vi "HandleObs.vi"(8 "error in (no error)":errorcluster, 11 "S4GUI in":refnum<class "S4GUI.lvclass">) -> (0 "error out":errorcluster, 3 "S4GUI out":refnum<class "S4GUI.lvclass">)   [LabVIEW 2018, in "S4GUI.lvclass"]
uses:
  S4GUI.lvclass
  S4GUI.lvclass/S4GUI.ctl
  Acquisition/Acquisition.lvclass
  Channel/Channel.lvclass
  StateMachine/State Machine.lvclass
  SyncBox/Sync Box.lvclass
  Trigger/Trigger.lvclass
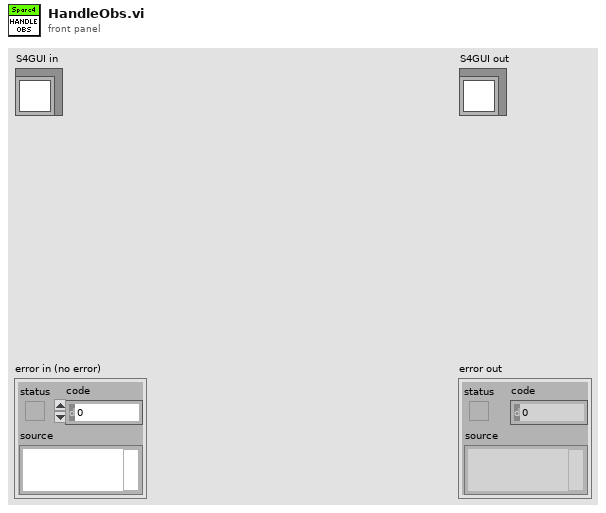
[diagram p1: front panel]
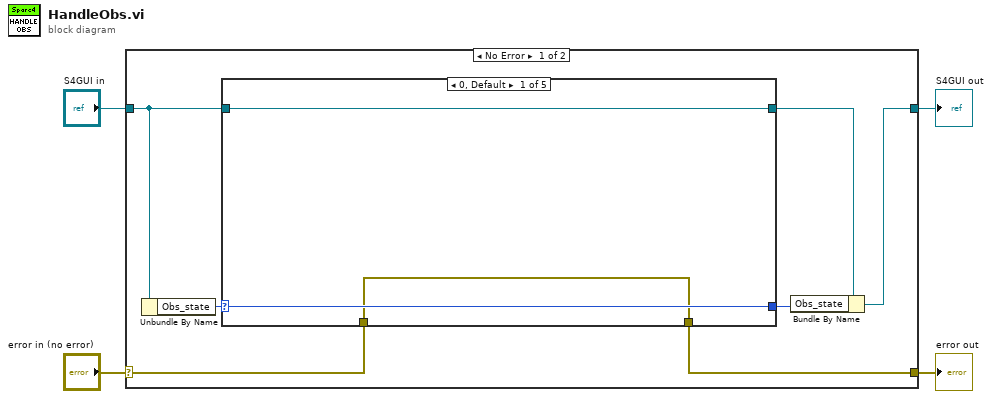
[diagram p0: block diagram]
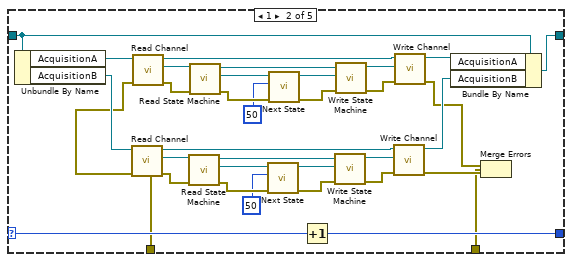
[diagram p2: hidden frame]
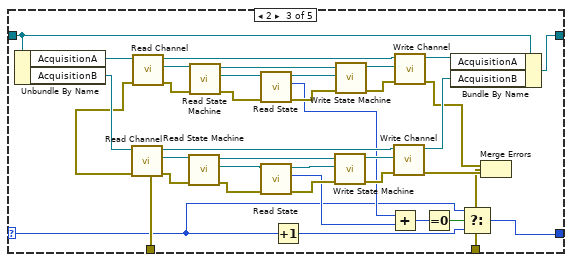
[diagram p3: hidden frame]
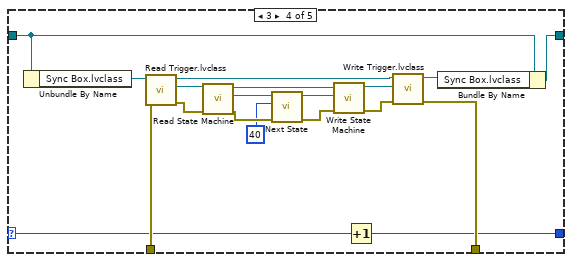
[diagram p4: hidden frame]
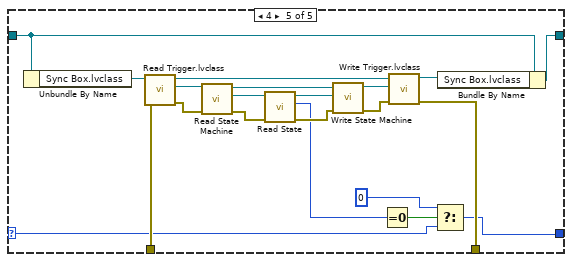
[diagram p5: hidden frame]
diagram:
  n1 = case shown="No Error" "error in (no error)" {
    selector: "error in (no error)" -> [w6 w127]
    tunnel: [w5 w127] -> w3
    tunnel: [w7 w126] -> w1
    tunnel: "S4GUI in" -> [w11 w126]
    frame No Error {
      n2 = Unbundle By Name(w11) -> ("Obs_state"=w10:u32)
      n3 = case shown="0, Default" w10 {
        selector: w10 -> [w14 w46 w49 w87 w109]
        tunnel: [w12 w48 w85 w104 w125] -> w9
        tunnel: w11 -> [w12 w47 w84 w103 w124]
        tunnel: [w14 w45 w50 w86 w105] -> w8
        tunnel: w6 -> [w13 w18 w67 w99 w120]
        tunnel: [w13 w15 w64 w98 w119] -> w5
        frame 0, Default {
        }
        frame 1 {
          n4 = Unbundle By Name(w47) -> ("AcquisitionA"=w44:refnum<class "Acquisition.lvclass">, "AcquisitionB"=w20:refnum<class "Acquisition.lvclass">)
          n5 = call-dynamic "Read Channel.vi"("error in (no error)"=w18, "Acquisition in"=w20) -> ("error out"=w30:errorcluster, "Channel.lvclass"=w29:refnum<class "Channel.lvclass">, "Acquisition out"=w31:refnum<class "Acquisition.lvclass">)  [unwired: 7 in]
          n6 = call-dynamic "Read Channel.vi"("error in (no error)"=w18, "Acquisition in"=w44) -> ("error out"=w41:errorcluster, "Channel.lvclass"=w40:refnum<class "Channel.lvclass">, "Acquisition out"=w42:refnum<class "Acquisition.lvclass">)  [unwired: 7 in]
          n7 = call-dynamic "Read State Machine.vi"("error in (no error)"=w30, "Device in"=w29) -> ("error out"=w25:errorcluster, "State Machine.lvclass"=w23:refnum<class "State Machine.lvclass">, "Device out"=w28:refnum<class "Channel.lvclass">)  [unwired: 7 in]
          n8 = call-dynamic "Read State Machine.vi"("error in (no error)"=w41, "Device in"=w40) -> ("error out"=w36:errorcluster, "State Machine.lvclass"=w34:refnum<class "State Machine.lvclass">, "Device out"=w39:refnum<class "Channel.lvclass">)  [unwired: 7 in]
          n9 = call "Next State.vi"("error in (no error)"=w25, "New_State"=50, "State Machine in"=w23) -> ("error out"=w21:errorcluster, "State Machine out"=w22:refnum<class "State Machine.lvclass">)  [unwired: 7 in]
          n10 = call "Next State.vi"("error in (no error)"=w36, "New_State"=50, "State Machine in"=w34) -> ("error out"=w32:errorcluster, "State Machine out"=w33:refnum<class "State Machine.lvclass">)  [unwired: 7 in]
          n11 = Increment(x=w46) -> (x+1=w45:u32)
          n12 = call-dynamic "Write State Machine.vi"("error in (no error)"=w21, "State Machine.lvclass"=w22, "Device in"=w28) -> ("error out"=w26:errorcluster, "Device out"=w27:refnum<class "Channel.lvclass">)  [unwired: 7 in]
          n13 = call-dynamic "Write State Machine.vi"("error in (no error)"=w32, "State Machine.lvclass"=w33, "Device in"=w39) -> ("error out"=w37:errorcluster, "Device out"=w38:refnum<class "Channel.lvclass">)  [unwired: 7 in]
          n14 = call-dynamic "Write Channel.vi"("error in (no error)"=w26, "Channel.lvclass"=w27, "Acquisition in"=w31) -> ("error out"=w16:errorcluster, "Acquisition out"=w19:refnum<class "Acquisition.lvclass">)  [unwired: 7 in]
          n15 = call-dynamic "Write Channel.vi"("error in (no error)"=w37, "Channel.lvclass"=w38, "Acquisition in"=w42) -> ("error out"=w17:errorcluster, "Acquisition out"=w43:refnum<class "Acquisition.lvclass">)  [unwired: 7 in]
          n16 = Bundle By Name(cluster=w47, "AcquisitionA"=w43, "AcquisitionB"=w19) -> (w48:refnum<class "S4GUI.lvclass">)
          n17 = Merge Errors(w17, w16) -> (w15:errorcluster)
        }
        frame 2 {
          n18 = Unbundle By Name(w84) -> ("AcquisitionA"=w83:refnum<class "Acquisition.lvclass">, "AcquisitionB"=w69:refnum<class "Acquisition.lvclass">)
          n19 = call-dynamic "Read Channel.vi"("error in (no error)"=w67, "Acquisition in"=w69) -> ("error out"=w74:errorcluster, "Channel.lvclass"=w73:refnum<class "Channel.lvclass">, "Acquisition out"=w75:refnum<class "Acquisition.lvclass">)  [unwired: 7 in]
          n20 = call-dynamic "Read Channel.vi"("error in (no error)"=w67, "Acquisition in"=w83) -> ("error out"=w80:errorcluster, "Channel.lvclass"=w79:refnum<class "Channel.lvclass">, "Acquisition out"=w81:refnum<class "Acquisition.lvclass">)  [unwired: 7 in]
          n21 = call-dynamic "Read State Machine.vi"("error in (no error)"=w74, "Device in"=w73) -> ("error out"=w57:errorcluster, "State Machine.lvclass"=w61:refnum<class "State Machine.lvclass">, "Device out"=w72:refnum<class "Channel.lvclass">)  [unwired: 7 in]
          n22 = call-dynamic "Read State Machine.vi"("error in (no error)"=w80, "Device in"=w79) -> ("error out"=w59:errorcluster, "State Machine.lvclass"=w63:refnum<class "State Machine.lvclass">, "Device out"=w78:refnum<class "Channel.lvclass">)  [unwired: 7 in]
          n23 = call-dynamic "Read State.vi"("error in (no error)"=w59, "State Machine in"=w63) -> ("error out"=w58:errorcluster, "State"=w55:i32, "State Machine out"=w62:refnum<class "State Machine.lvclass">)  [unwired: 7 in]
          n24 = call-dynamic "Read State.vi"("error in (no error)"=w57, "State Machine in"=w61) -> ("error out"=w56:errorcluster, "State"=w54:i32, "State Machine out"=w60:refnum<class "State Machine.lvclass">)  [unwired: 7 in]
          n25 = Increment(x=w49) -> (x+1=w51:u32)
          n26 = call-dynamic "Write State Machine.vi"("error in (no error)"=w56, "State Machine.lvclass"=w60, "Device in"=w72) -> ("error out"=w70:errorcluster, "Device out"=w71:refnum<class "Channel.lvclass">)  [unwired: 7 in]
          n27 = call-dynamic "Write State Machine.vi"("error in (no error)"=w58, "State Machine.lvclass"=w62, "Device in"=w78) -> ("error out"=w76:errorcluster, "Device out"=w77:refnum<class "Channel.lvclass">)  [unwired: 7 in]
          n28 = Add(x=w55, y=w54) -> (x+y=w53:i32)
          n29 = call-dynamic "Write Channel.vi"("error in (no error)"=w70, "Channel.lvclass"=w71, "Acquisition in"=w75) -> ("error out"=w65:errorcluster, "Acquisition out"=w68:refnum<class "Acquisition.lvclass">)  [unwired: 7 in]
          n30 = call-dynamic "Write Channel.vi"("error in (no error)"=w76, "Channel.lvclass"=w77, "Acquisition in"=w81) -> ("error out"=w66:errorcluster, "Acquisition out"=w82:refnum<class "Acquisition.lvclass">)  [unwired: 7 in]
          n31 = Equal To 0?(x=w53) -> (x = 0?=w52:bool)
          n32 = Bundle By Name(cluster=w84, "AcquisitionA"=w82, "AcquisitionB"=w68) -> (w85:refnum<class "S4GUI.lvclass">)
          n33 = Select(t=w49, s=w52, f=w51) -> (s? t:f=w50:u32)
          n34 = Merge Errors(w66, w65) -> (w64:errorcluster)
        }
        frame 3 {
          n35 = Unbundle By Name(w103) -> ("Sync Box.lvclass"=w102:refnum<class "Sync Box.lvclass">)
          n36 = call-dynamic "Read Trigger.lvclass.vi"("error in (no error)"=w99, "Sync Box in"=w102) -> ("error out"=w97:errorcluster, "Trigger.lvclass"=w96:refnum<class "Trigger.lvclass">, "Sync Box out"=w100:refnum<class "Sync Box.lvclass">)  [unwired: 7 in]
          n37 = call-dynamic "Read State Machine.vi"("error in (no error)"=w97, "Device in"=w96) -> ("error out"=w92:errorcluster, "State Machine.lvclass"=w90:refnum<class "State Machine.lvclass">, "Device out"=w95:refnum<class "Trigger.lvclass">)  [unwired: 7 in]
          n38 = call "Next State.vi"("error in (no error)"=w92, "New_State"=40, "State Machine in"=w90) -> ("error out"=w88:errorcluster, "State Machine out"=w89:refnum<class "State Machine.lvclass">)  [unwired: 7 in]
          n39 = call-dynamic "Write State Machine.vi"("error in (no error)"=w88, "State Machine.lvclass"=w89, "Device in"=w95) -> ("error out"=w93:errorcluster, "Device out"=w94:refnum<class "Trigger.lvclass">)  [unwired: 7 in]
          n40 = Increment(x=w87) -> (x+1=w86:u32)
          n41 = call-dynamic "Write Trigger.lvclass.vi"("error in (no error)"=w93, "Trigger.lvclass"=w94, "Sync Box in"=w100) -> ("error out"=w98:errorcluster, "Sync Box out"=w101:refnum<class "Sync Box.lvclass">)  [unwired: 7 in]
          n42 = Bundle By Name(cluster=w103, "Sync Box.lvclass"=w101) -> (w104:refnum<class "S4GUI.lvclass">)
        }
        frame 4 {
          n43 = Unbundle By Name(w124) -> ("Sync Box.lvclass"=w123:refnum<class "Sync Box.lvclass">)
          n44 = call-dynamic "Read Trigger.lvclass.vi"("error in (no error)"=w120, "Sync Box in"=w123) -> ("error out"=w118:errorcluster, "Trigger.lvclass"=w117:refnum<class "Trigger.lvclass">, "Sync Box out"=w121:refnum<class "Sync Box.lvclass">)  [unwired: 7 in]
          n45 = call-dynamic "Read State Machine.vi"("error in (no error)"=w118, "Device in"=w117) -> ("error out"=w111:errorcluster, "State Machine.lvclass"=w113:refnum<class "State Machine.lvclass">, "Device out"=w116:refnum<class "Trigger.lvclass">)  [unwired: 7 in]
          n46 = call-dynamic "Read State.vi"("error in (no error)"=w111, "State Machine in"=w113) -> ("error out"=w110:errorcluster, "State"=w106:i32, "State Machine out"=w112:refnum<class "State Machine.lvclass">)  [unwired: 7 in]
          n47 = call-dynamic "Write State Machine.vi"("error in (no error)"=w110, "State Machine.lvclass"=w112, "Device in"=w116) -> ("error out"=w114:errorcluster, "Device out"=w115:refnum<class "Trigger.lvclass">)  [unwired: 7 in]
          n48 = Equal To 0?(x=w106) -> (x = 0?=w107:bool)
          n49 = call-dynamic "Write Trigger.lvclass.vi"("error in (no error)"=w114, "Trigger.lvclass"=w115, "Sync Box in"=w121) -> ("error out"=w119:errorcluster, "Sync Box out"=w122:refnum<class "Sync Box.lvclass">)  [unwired: 7 in]
          n50 = Select(t=u32 0 ("Obs_state"), s=w107, f=w109) -> (s? t:f=w105:u32)
          n51 = Bundle By Name(cluster=w124, "Sync Box.lvclass"=w122) -> (w125:refnum<class "S4GUI.lvclass">)
        }
      }
      n52 = Bundle By Name(cluster=w9, "Obs_state"=w8) -> (w7:refnum<class "S4GUI.lvclass">)
    }
    frame Error {
    }
  }
  "error out" <- w3
  "S4GUI out" <- w1
